vi "uService not responding.vi"(8 "error in (no error)":errorcluster, 10 "uService":string, 11 "Guardian in":refnum<class "Guardian.lvclass">) -> (0 "error out":errorcluster, 3 "Guardian out":refnum<class "Guardian.lvclass">)   [LabVIEW 2026, in "TALOS.lvlib" / "Guardian.lvlib" / "Guardian.lvclass"]
uses:
  Guardian.lvclass
  C:/LabVIEW Code/TALOS/builds/Actor Framework PPL/Actor Framework.lvlibp/1abvi3w/vi.lib/ActorFramework/Actor/Actor.lvclass
  Guardian.lvclass/Guardian.ctl
  Ancestor/Ancestor/Ancestor.lvclass/Ancestor.ctl
  Guardian Messages/Kill uService Msg/Kill uService Msg.lvclass/Kill uService Msg.ctl
  ec96dbe9-becf-4abc-a5c2-614e58e26ee7.vi
  FGV/Error Memory/Get Error Description.vi
  Support VIs/Get PC name.vi
  Ancestor/Ancestor/Read ID.vi
  Support VIs/Get Class Name.vi
  <vilib>/Utility/error.llb/Clear Errors.vi
  FGV/Error Memory/Error Memory Core.vi
  <vilib>/AdvancedString/Delimited String to 1D String Array.vi
  <vilib>/AdvancedString/Delimited String to 1D String Array (string).vi
  Support VIs/Circus Root Path.vi
  FGV/Error Memory/Error Crt Lvl checker.vi
  FGV/Error Memory/Error Memory Core.vi/40c8088d-b597-4017-91af-faa98e00292e.vi
  FGV/Error Memory/Error Memory Core.vi/d4a3ab98-063c-4e44-b43d-fbdcfe6c2be2.vi
  Support VIs/Global Memory.vi
  <vilib>/Utility/LVClass/Get LV Class Name.vi
  Support VIs/Is in Packed Library.vi
  Support VIs/TALOS Root path.vi
  Support VIs/Read CSV worksheet.vi
  Support VIs/Global Constants.vi
  <vilib>/Utility/error.llb/General Error Handler.vi
  builds/Actor Framework PPL/Actor Framework.lvlibp/1abvi3w/vi.lib/ActorFramework/Message Enqueuer/Enqueue.vi
  Support VIs/Error Log.vi
  <vilib>/Comparison/Equal/Equal Functor/Equal Functor.lvclass
  Ancestor/Ancestor/Ancestor.lvclass
  Guardian Messages/Kill uService Msg/Kill uService Msg.lvclass
  TALOS.lvlib
  builds/Actor Framework PPL/Actor Framework.lvlibp/1abvi3w/vi.lib/ActorFramework/Actor/Actor.lvclass
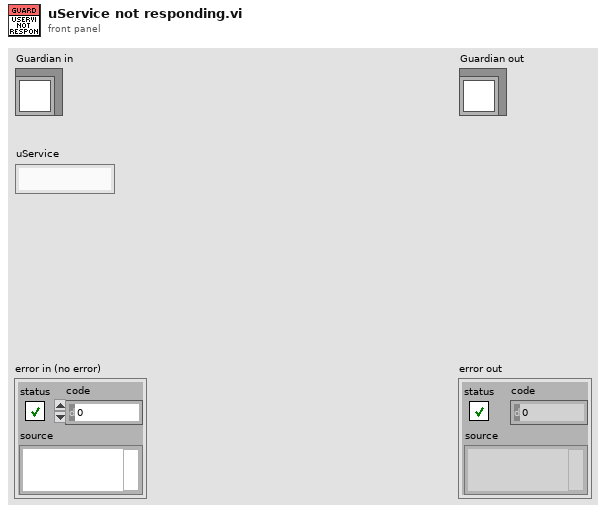
[diagram p1: front panel]
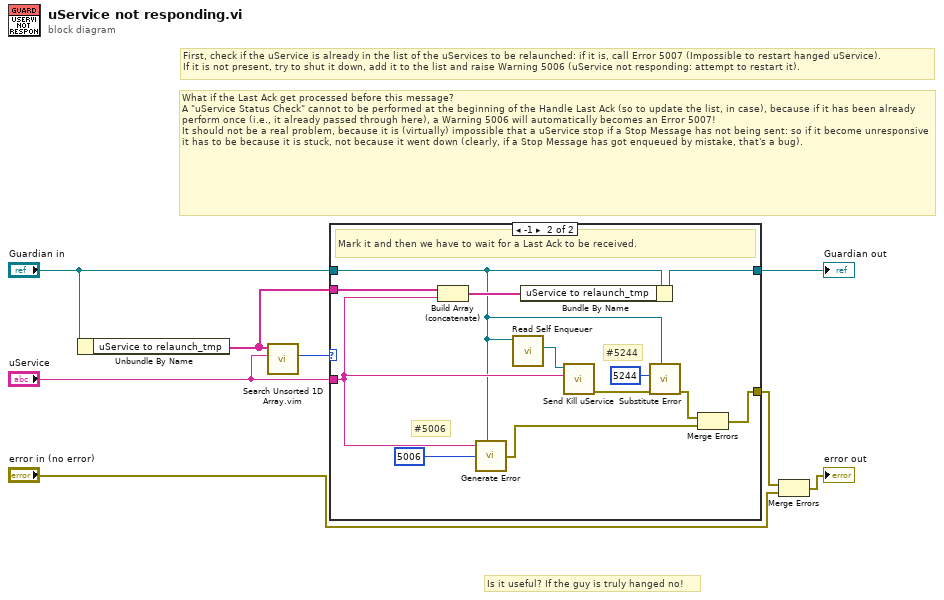
[diagram p0: block diagram]
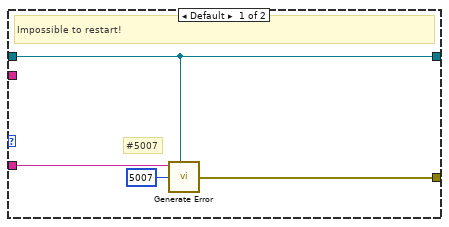
[diagram p2: hidden frame]
diagram:
  # "Is it useful? If the guy is truly hanged no!"
  # "First, check if the uService is already in the list of the uServices to be relaunched: if it is, call Error 5007 (Impossible to restart hanged uService).\nIf it is not present, try to shut it down, add it to the list and raise Warning 5006 (uService not responding: attempt to restart it)."
  # "What if the Last Ack get processed before this message? \nA \"uService Status Check\" cannot to be performed at the beginning of the Handle Last Ack (so to update the list, in case), because if it has been already perform once (i.e., it already passed through here), a Warning 5006 will automatically becomes an Error 5007!\nIt should not be a real problem, because it is (virtually) impossible that a uService stop if a Stop Message has not being sent: so if it become unresponsive it has to be because it is stuck, not because it went down (clearly, if a Stop Message has got enqueued by mistake, that's a bug)."
  n1 = Unbundle By Name("Guardian in") -> ("uService to relaunch_tmp"=w3:string[])
  n2 = call "Search Unsorted 1D Array.vim"("element"="uService", "unsorted 1D array"=w3) -> ("index of element"=w7:i32)  [unwired: 9 in]
  n3 = case shown="-1" w7 {
    tunnel: "uService" -> [w11 w19]
    tunnel: "Guardian in" -> [w10 w13]
    tunnel: [w10 w24] -> w4
    tunnel: w3 -> [_ w23]
    tunnel: [w9 w17] -> w2
    frame Default {
      # "#5007"
      # "Impossible to restart!"
      n4 = call "Generate Error.vi"("Optional String"=w11, "Class"=w10, "Error Code"=5007) -> ("error out"=w9:errorcluster)  [unwired: 4 in]
    }
    frame -1 {
      # "#5244"
      # "#5006"
      # "Mark it and then we have to wait for a Last Ack to be received."
      n5 = Build Array (concatenate)(w23, w19) -> (w22:string[])
      n6 = call "Generate Error.vi"("Optional String"=w19, "Class"=w13, "Error Code"=5006) -> ("error out"=w20:errorcluster)  [unwired: 4 in]
      n7 = call "Read Self Enqueuer.vi"("Actor"=w13) -> ("Self Enqueuer"=w18:refnum<class "Message Enqueuer.lvclass">)  [unwired: 10 in]
      n8 = Bundle By Name(cluster=w13, "uService to relaunch_tmp"=w22) -> (w24:refnum<class "Guardian.lvclass">)
      n9 = call "Send Kill uService.vi"("uService"=w19, "Message Enqueuer"=w18) -> ("error out"=w15:errorcluster)  [unwired: 8 in, 1 out]
      n10 = call "Substitute Error.vi"("LabVIEW Object"=w13, "error in (no error)"=w15, "Error Code"=5244) -> ("error out"=w14:errorcluster)  [unwired: 8 in]
      n11 = Merge Errors(w14, w20) -> (w17:errorcluster)
    }
  }
  "Guardian out" <- w4
  n12 = Merge Errors(w2, "error in (no error)") -> (→"error out":errorcluster)
